vi "passDataLoop2array.vi"() -> ()   [LabVIEW 2020]
uses:
  <vilib>/Waveform/DWDTOps.llb/DWDT Analog to Digital.vi
panel:
  out "x/y":dbl
  out "digital waveform":digitalwaveform(waveform)={"t0"=timestamp(0 s since 1904-01-01), "dt"=0.0, "Y"={"transitions"=[], "data"=[]}, "error"={"status"=FALSE, "code"=37421928, "source"=""}}
  out "XY Graph 2":cluster{i32[], dbl[]}(graph)
  out "XY Graph":cluster{i32[], dbl[]}(graph)
  in  "Tab Control":enum32{"Page 1", "Page 2"}(tab)
  out "digital signal 2":bool[](array[boolean])
  in  "initial value":dbl
  in  "value":bool
  in  "final value":dbl
  out "i":i32
  out "Array 2":bool[](array[boolean]) caption="digital signal"
  out "Analog_signal":dbl
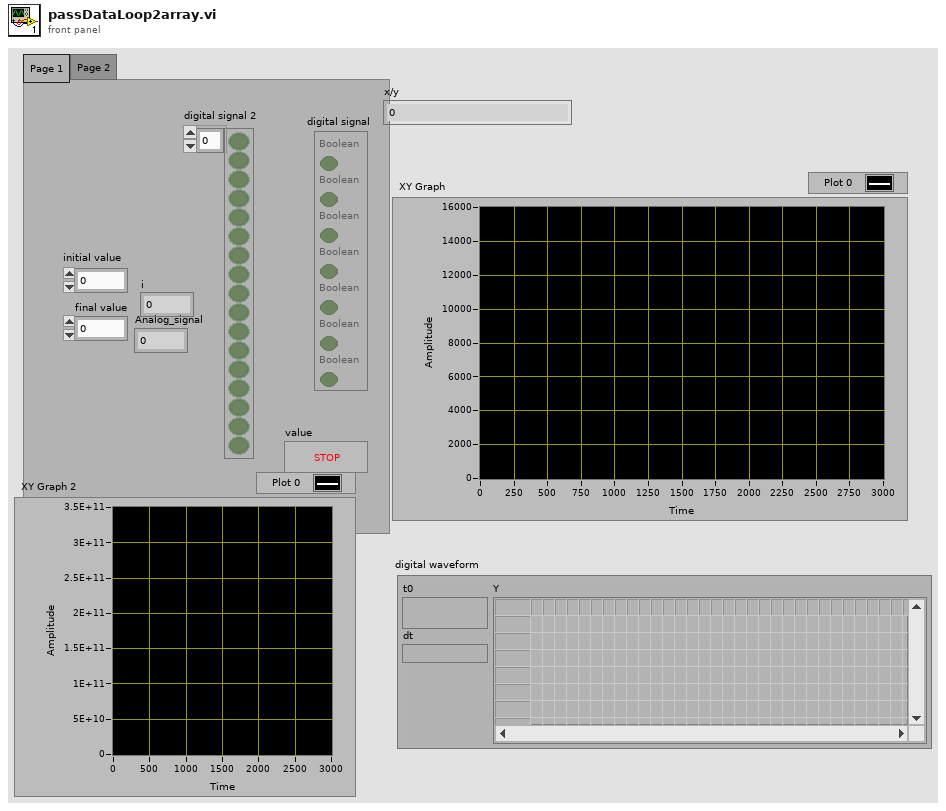
[diagram p1: front panel]
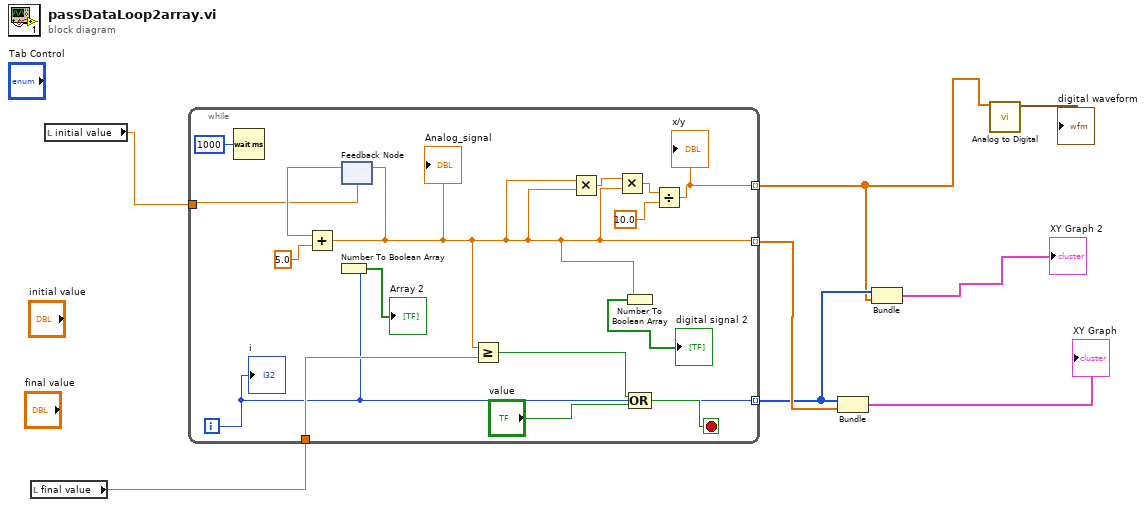
[diagram p0: block diagram]
diagram:
  n1 = local read "final value"() -> (w8:dbl)
  n2 = local read "initial value"() -> (w7:dbl)
  n3 = while {
    tunnel: w8 -> [w21]
    tunnel: w7 -> [w18]
    tunnel: [w12] -> w6 mode=indexing
    tunnel: [w9] -> w3 mode=indexing
    tunnel: [w15] -> w2 mode=indexing
    i -> [w9]
    stop <- w24 stop-if-true
    n4 = Wait (ms)(milliseconds to wait=u32 1000) -> ()  [unwired: 1 out]
    n5 = Number To Boolean Array(number=w9) -> (Boolean array=→"Array 2":bool[])
    n6 = feedback #1(w18) -> (w19:dbl)
    n7 = Add(x=w19, y=5.0) -> (x+y=w12:dbl)
    "Analog_signal" <- w12
    n8 = feedback-in #1(w12) -> ()
    n9 = Greater Or Equal?(x=w12, y=w21) -> (x >= y?=w22:bool)
    n10 = Multiply(x=w12, y=w12) -> (x*y=w13:dbl)
    n11 = Multiply(x=w13, y=w12) -> (x*y=w14:dbl)
    n12 = Number To Boolean Array(number=w12) -> (Boolean array=→"digital signal 2":bool[])
    n13 = Compound Arithmetic op=OR(w22, "value") -> (w24:bool)
    n14 = Divide(x=w14, y=10.0) -> (x/y=w15:dbl)
    "x/y" <- w15
    "i" <- w9
  }
  n15 = Bundle(w3, w6) -> (→"XY Graph":cluster{i32[], dbl[]})  [unwired: 1 in]
  n16 = Bundle(w3, w2) -> (→"XY Graph 2":cluster{i32[], dbl[]})  [unwired: 1 in]
  n17 = call-poly <vilib>:"Analog to Digital.vi"("analog waveform"=w2) -> ("digital waveform"=→"digital waveform":digitalwaveform)  [unwired: 7 in, 3 out]
